vi "newMain.vi"() -> ()   [LabVIEW 2013]
uses:
  <vilib>/NXT/Block Support/NXT_InputPort.ctl
  <vilib>/NXT/Block Support/NXT_OutputPort.ctl
  <vilib>/NXT/Dual Mode Library/Sensors/EV3_Gyro_Reset.vi
  <vilib>/NXT/Dual Mode Library/Sensors/EV3_Ultrasonic_CM.vi
  <vilib>/NXT/NXTIO Xnodes/NXTIONodeSubVIs/NXTStopMotors.vi
  <vilib>/NXT/Subs/LVHSConnector.ctl
  <vilib>/NXT/NXTIO Xnodes/AddressXNode/NXTIOAddress.xnode
  <vilib>/NXT/NXTIO Xnodes/NXTIOXNode/NXTIO.xnode
  <vilib>/NXT/LegoClasses/BrickReference/BrickReference.lvclass
panel:
  out "Numeric 3":dbl
  out "Numeric 2":dbl
  out "Numeric":dbl
  out "isWhite 2":bool
  out "Whiteandblack":bool
  out "blackandwhite":bool
  out "Boolean":bool
  out "to_change":bool
  out "x <= y?":bool
  out "isWhite":bool
  out "isBlack":bool
  out "BlackThenWhite":bool
  out "leftA":dbl
  out "rightB":dbl
  out "identificationWhite":dbl
  out "numOfTargil":dbl
  out "identificationBlack":dbl
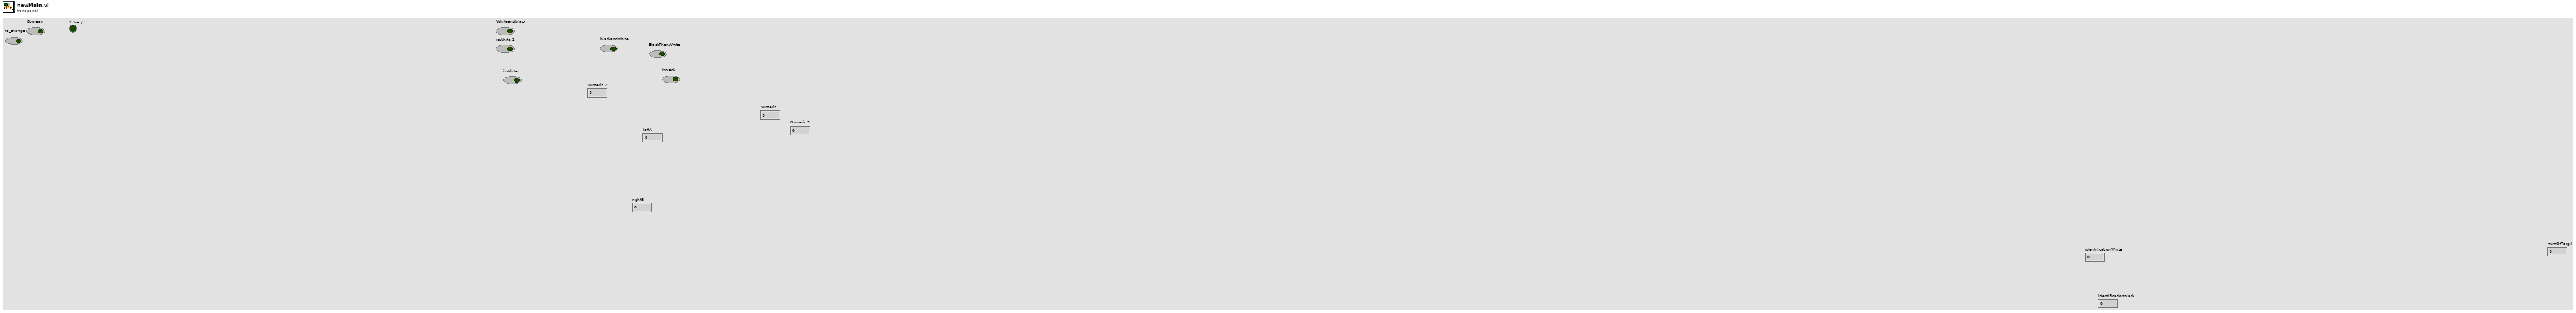
[diagram p1: front panel]
types:
  T1 = typedef "NXT_OutputPort.ctl" = u8
  T2 = typedef "NXT_InputPort.ctl" = u32
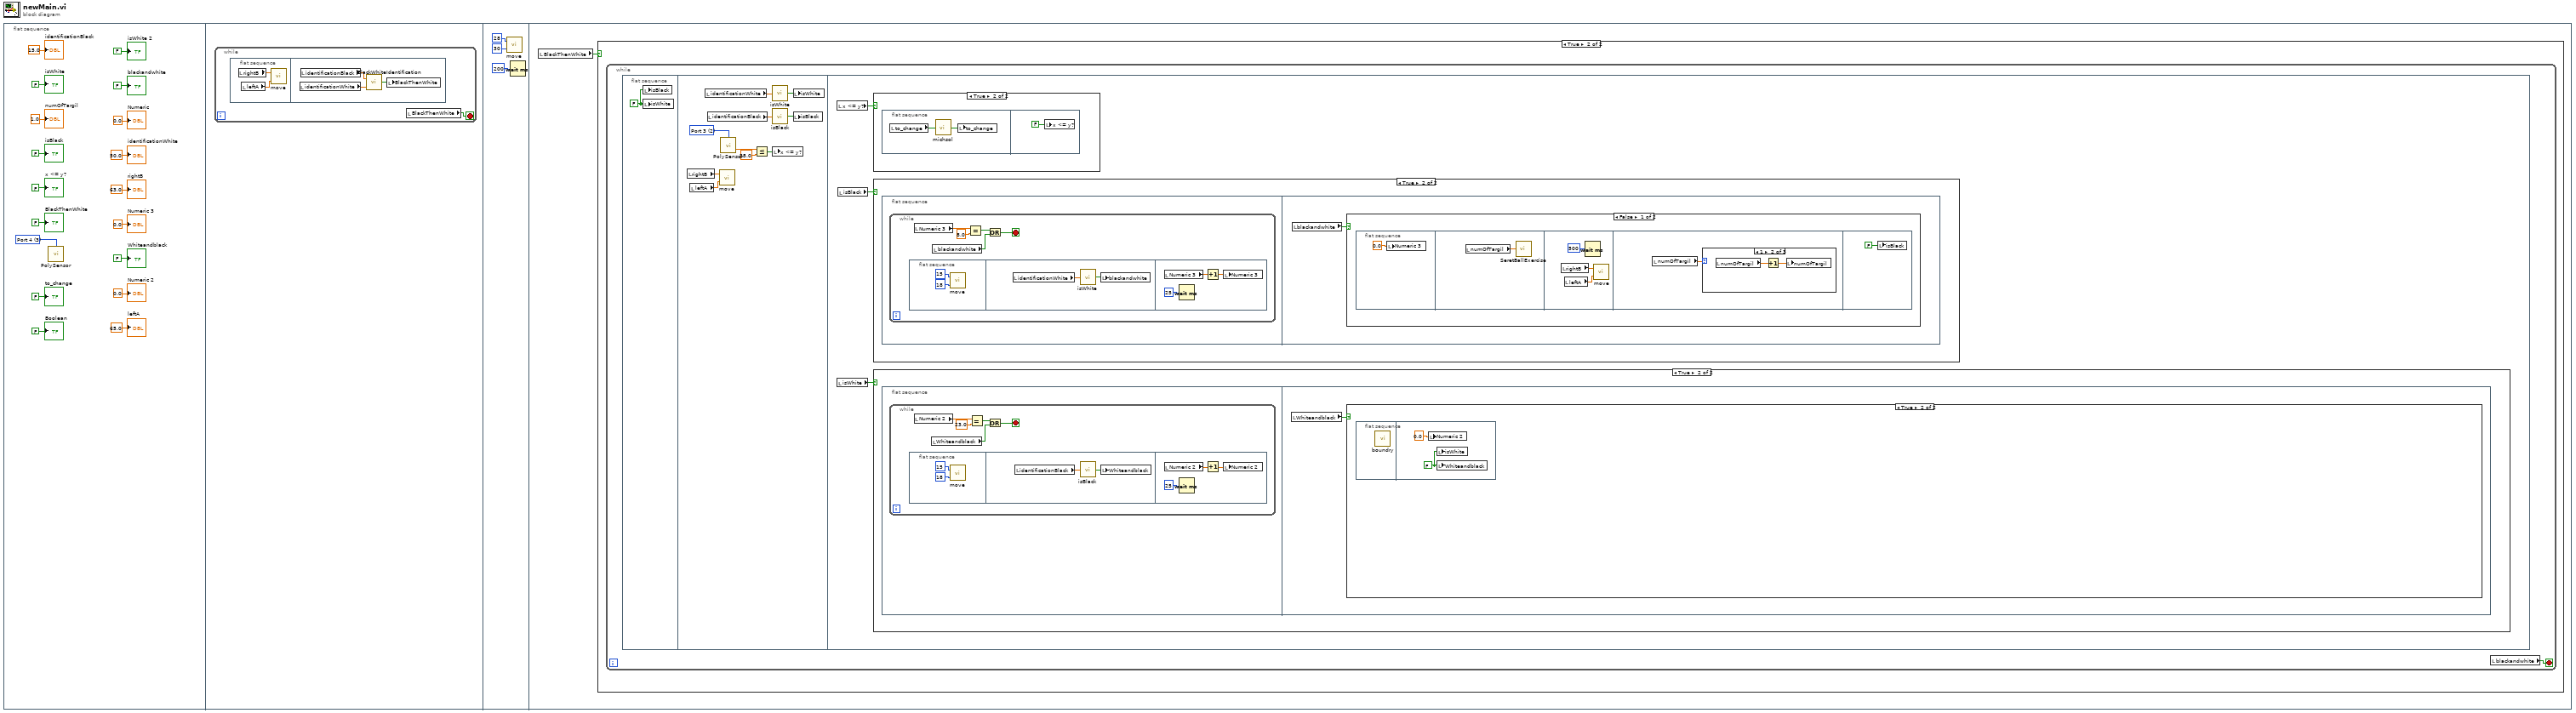
[diagram p0: block diagram]
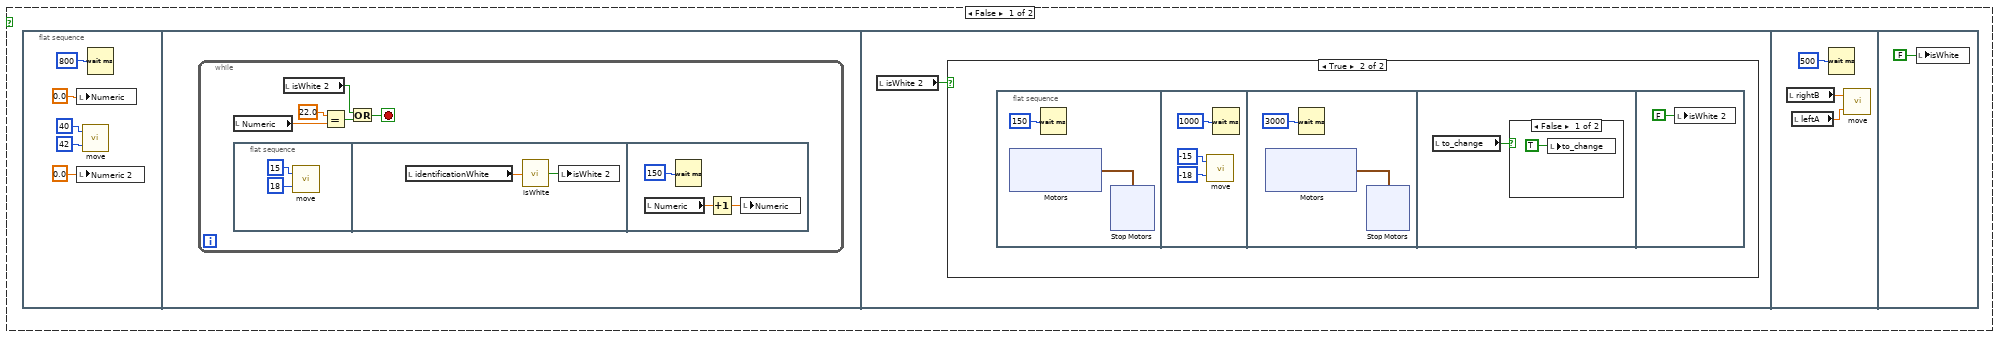
[diagram p4: hidden frame]
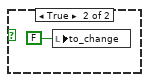
[diagram p6: hidden frame]
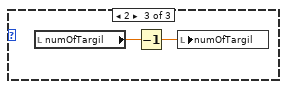
[diagram p9: hidden frame]
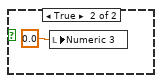
[diagram p10: hidden frame]
diagram:
  n1 = flat-sequence {
    frame #0 {
      w13 = T2 3 items=["Port 1", "Port 2", "Port 3", "Port 4"] ("Port (Port 1)")
      n2 = call-poly <vilib>:"PolySensor.vi"("Port (Port 1)"=w13) -> ()  [unwired: 3 in, 1 out]
      "identificationBlack" <- 15.0 ("identificationBlack")
      "numOfTargil" <- 1.0 ("numOfTargil")
      "identificationWhite" <- 50.0 ("identificationWhite")
      "rightB" <- 63.0 ("Numeric")
      "leftA" <- 65.0 ("leftA")
      "x <= y?" <- FALSE ("x <= y?")
      "isBlack" <- FALSE ("isBlack")
      "isWhite" <- FALSE ("isWhite")
      "to_change" <- FALSE ("Boolean")
      "Boolean" <- FALSE ("Boolean")
      "blackandwhite" <- FALSE ("blackandwhite")
      "Whiteandblack" <- FALSE ("Whiteandblack")
      "BlackThenWhite" <- FALSE ("BlackThenWhite")
      "isWhite 2" <- FALSE ("isWhite 2")
      "Numeric" <- 0.0 ("Numeric")
      "Numeric 2" <- 0.0 ("Numeric 2")
      "Numeric 3" <- 0.0 ("Numeric 3")
    }
    frame #1 {
      n3 = while {
        stop <- w19 stop-if-true
        n4 = flat-sequence {
          frame #0 {
            n5 = local read "rightB"() -> (w20:dbl)
            n6 = local read "leftA"() -> (w21:dbl)
            n7 = call "move.vi"("speedLeft"=w21, "speedRight"=w20) -> ()  [unwired: 1 in]
          }
          frame #1 {
            n8 = local read "identificationWhite"() -> (w23:dbl)
            n9 = local read "identificationBlack"() -> (w24:dbl)
            n10 = call "BlackWhiteIdentification.vi"("whiteBOND"=w23, "BlackBOND"=w24) -> ("BlackThenWhite"=w22:bool)
            n11 = local write "BlackThenWhite"(w22) -> ()
          }
        }
        n12 = local read "BlackThenWhite"() -> (w19:bool)
      }
    }
    frame #2 {
      n13 = call "move.vi"("speedLeft"=i8 30, "speedRight"=i8 28) -> ()  [unwired: 1 in]
      n14 = Wait (ms)(milliseconds to wait=u32 200) -> ()  [unwired: 1 out]
    }
    frame #3 {
      n15 = local read "BlackThenWhite"() -> (w28:bool)
      n16 = case shown="True" w28 {
        frame False {
        }
        frame True {
          n17 = while {
            stop <- w29 stop-if-true
            n18 = flat-sequence {
              frame #0 {
                w30 = FALSE ("isBlack")
                n19 = local write "isBlack"(w30) -> ()
                n20 = local write "isWhite"(w30) -> ()
              }
              frame #1 {
                w39 = T2 2 items=["Port 1", "Port 2", "Port 3", "Port 4"] ("Port (Port 1)")
                n21 = local read "rightB"() -> (w36:dbl)
                n22 = local read "leftA"() -> (w35:dbl)
                n23 = local read "identificationWhite"() -> (w40:dbl)
                n24 = local read "identificationBlack"() -> (w32:dbl)
                n25 = call "move.vi"("speedLeft"=w35, "speedRight"=w36) -> ()  [unwired: 1 in]
                n26 = call-poly <vilib>:"PolySensor.vi"("Port (Port 1)"=w39) -> ("Centimeters"=w38:sgl)  [unwired: 2 in, 1 out]
                n27 = Less Or Equal?(x=w38, y=sgl 35.0) -> (x <= y?=w34:bool)
                n28 = call "isWhite.vi"("whiteBOND"=w40) -> ("isWhite"=w33:bool)
                n29 = call "isBlack.vi"("BlackBOND"=w32) -> ("isBlack"=w31:bool)
                n30 = local write "x <= y?"(w34) -> ()
                n31 = local write "isWhite"(w33) -> ()
                n32 = local write "isBlack"(w31) -> ()
              }
              frame #2 {
                n33 = local read "x <= y?"() -> (w43:bool)
                n34 = local read "isWhite"() -> (w41:bool)
                n35 = local read "isBlack"() -> (w42:bool)
                n36 = case shown="True" w43 {
                  frame False {
                  }
                  frame True {
                    n37 = flat-sequence {
                      frame #0 {
                        n38 = local read "to_change"() -> (w130:bool)
                        n39 = call "michsol.vi"("LEFTOTRETE"=w130) -> ("Boolean"=w129:bool)
                        n40 = local write "to_change"(w129) -> ()
                      }
                      frame #1 {
                        n41 = local write "x <= y?"(FALSE ("x <= y?")) -> ()
                      }
                    }
                  }
                }
                n42 = case shown="True" w42 {
                  frame False {
                  }
                  frame True {
                    n43 = flat-sequence {
                      frame #0 {
                        n44 = while {
                          stop <- w104 stop-if-true
                          n45 = flat-sequence {
                            frame #0 {
                              n46 = call "move.vi"("speedLeft"=i8 18, "speedRight"=i8 15) -> ()  [unwired: 1 in]
                            }
                            frame #1 {
                              n47 = local read "identificationWhite"() -> (w111:dbl)
                              n48 = call "isWhite.vi"("whiteBOND"=w111) -> ("isWhite"=w112:bool)
                              n49 = local write "blackandwhite"(w112) -> ()
                            }
                            frame #2 {
                              n50 = local read "Numeric 3"() -> (w114:dbl)
                              n51 = Wait (ms)(milliseconds to wait=u32 25) -> ()  [unwired: 1 out]
                              n52 = Increment(x=w114) -> (x+1=w115:dbl)
                              n53 = local write "Numeric 3"(w115) -> ()
                            }
                          }
                          n54 = local read "Numeric 3"() -> (w105:dbl)
                          n55 = local read "blackandwhite"() -> (w107:bool)
                          n56 = Equal?(x=w105, y=8.0) -> (x = y?=w106:bool)
                          n57 = Or(x=w106, y=w107) -> (x .or. y?=w104:bool)
                        }
                      }
                      frame #1 {
                        n58 = local read "blackandwhite"() -> (w116:bool)
                        n59 = case shown="False" w116 {
                          frame False {
                            n60 = flat-sequence {
                              frame #0 {
                                n61 = local write "Numeric 3"(0.0 ("Numeric 3")) -> ()
                              }
                              frame #1 {
                                n62 = local read "numOfTargil"() -> (w118:dbl)
                                n63 = call "SeretBallExercise.vi"("ROUND"=w118) -> ()  [unwired: 1 in]
                              }
                              frame #2 {
                                n64 = local read "rightB"() -> (w120:dbl)
                                n65 = local read "leftA"() -> (w119:dbl)
                                n66 = Wait (ms)(milliseconds to wait=u32 500) -> ()  [unwired: 1 out]
                                n67 = call "move.vi"("speedLeft"=w119, "speedRight"=w120) -> ()  [unwired: 1 in]
                              }
                              frame #3 {
                                n68 = local read "numOfTargil"() -> (w122:dbl)
                                n69 = case shown="1" w122 {
                                frame 0, Default {
                                }
                                frame 1 {
                                n70 = local read "numOfTargil"() -> (w124:dbl)
                                n71 = Increment(x=w124) -> (x+1=w123:dbl)
                                n72 = local write "numOfTargil"(w123) -> ()
                                }
                                frame 2 {
                                n73 = local read "numOfTargil"() -> (w126:dbl)
                                n74 = Decrement(x=w126) -> (x-1=w125:dbl)
                                n75 = local write "numOfTargil"(w125) -> ()
                                }
                                }
                              }
                              frame #4 {
                                n76 = local write "isBlack"(FALSE ("isBlack")) -> ()
                              }
                            }
                          }
                          frame True {
                            n77 = local write "Numeric 3"(0.0 ("Numeric 3")) -> ()
                          }
                        }
                      }
                    }
                  }
                }
                n78 = case shown="True" w41 {
                  frame False {
                  }
                  frame True {
                    n79 = flat-sequence {
                      frame #0 {
                        n80 = while {
                          stop <- w45 stop-if-true
                          n81 = flat-sequence {
                            frame #0 {
                              n82 = call "move.vi"("speedLeft"=i8 18, "speedRight"=i8 15) -> ()  [unwired: 1 in]
                            }
                            frame #1 {
                              n83 = local read "identificationBlack"() -> (w52:dbl)
                              n84 = call "isBlack.vi"("BlackBOND"=w52) -> ("isBlack"=w51:bool)
                              n85 = local write "Whiteandblack"(w51) -> ()
                            }
                            frame #2 {
                              n86 = local read "Numeric 2"() -> (w55:dbl)
                              n87 = Wait (ms)(milliseconds to wait=u32 25) -> ()  [unwired: 1 out]
                              n88 = Increment(x=w55) -> (x+1=w54:dbl)
                              n89 = local write "Numeric 2"(w54) -> ()
                            }
                          }
                          n90 = local read "Numeric 2"() -> (w48:dbl)
                          n91 = local read "Whiteandblack"() -> (w46:bool)
                          n92 = Equal?(x=w48, y=23.0) -> (x = y?=w47:bool)
                          n93 = Or(x=w47, y=w46) -> (x .or. y?=w45:bool)
                        }
                      }
                      frame #1 {
                        n94 = local read "Whiteandblack"() -> (w56:bool)
                        n95 = case shown="True" w56 {
                          frame False {
                            n96 = flat-sequence {
                              frame #0 {
                                n97 = local write "Numeric"(0.0 ("Numeric")) -> ()
                                n98 = local write "Numeric 2"(0.0 ("Numeric 2")) -> ()
                                n99 = call "move.vi"("speedLeft"=i8 42, "speedRight"=i8 40) -> ()  [unwired: 1 in]
                                n100 = Wait (ms)(milliseconds to wait=u32 800) -> ()  [unwired: 1 out]
                              }
                              frame #1 {
                                n101 = while {
                                stop <- w65 stop-if-true
                                n102 = local read "Numeric"() -> (w63:dbl)
                                n103 = flat-sequence {
                                frame #0 {
                                n104 = call "move.vi"("speedLeft"=i8 18, "speedRight"=i8 15) -> ()  [unwired: 1 in]
                                }
                                frame #1 {
                                n105 = local read "identificationWhite"() -> (w70:dbl)
                                n106 = call "isWhite.vi"("whiteBOND"=w70) -> ("isWhite"=w69:bool)
                                n107 = local write "isWhite 2"(w69) -> ()
                                }
                                frame #2 {
                                n108 = local read "Numeric"() -> (w73:dbl)
                                n109 = Wait (ms)(milliseconds to wait=u32 150) -> ()  [unwired: 1 out]
                                n110 = Increment(x=w73) -> (x+1=w72:dbl)
                                n111 = local write "Numeric"(w72) -> ()
                                }
                                }
                                n112 = local read "isWhite 2"() -> (w66:bool)
                                n113 = Equal?(x=22.0, y=w63) -> (x = y?=w62:bool)
                                n114 = Or(x=w66, y=w62) -> (x .or. y?=w65:bool)
                                }
                              }
                              frame #2 {
                                n115 = local read "isWhite 2"() -> (w74:bool)
                                n116 = case shown="True" w74 {
                                frame False {
                                }
                                frame True {
                                n117 = flat-sequence {
                                frame #0 {
                                n118 = xnode "Motors"() -> ("Motor"=w76:cluster{"Port":T1, "Port":T1})
                                n119 = Wait (ms)(milliseconds to wait=u32 150) -> ()  [unwired: 1 out]
                                n120 = xnode "Stop Motors"("Motors"=w76) -> ()  [unwired: 1 in, 1 out]
                                }
                                frame #1 {
                                n121 = call "move.vi"("speedLeft"=i8 -18, "speedRight"=i8 -15) -> ()  [unwired: 1 in]
                                n122 = Wait (ms)(milliseconds to wait=u32 1000) -> ()  [unwired: 1 out]
                                }
                                frame #2 {
                                n123 = xnode "Motors"() -> ("Motor"=w87:cluster{"Port":T1, "Port":T1})
                                n124 = Wait (ms)(milliseconds to wait=u32 3000) -> ()  [unwired: 1 out]
                                n125 = xnode "Stop Motors"("Motors"=w87) -> ()  [unwired: 1 in, 1 out]
                                }
                                frame #3 {
                                n126 = local read "to_change"() -> (w94:bool)
                                n127 = case shown="False" w94 {
                                frame False {
                                n128 = local write "to_change"(TRUE ("to_change")) -> ()
                                }
                                frame True {
                                n129 = local write "to_change"(FALSE ("to_change")) -> ()
                                }
                                }
                                }
                                frame #4 {
                                n130 = local write "isWhite 2"(FALSE ("isWhite 2")) -> ()
                                }
                                }
                                }
                                }
                              }
                              frame #3 {
                                n131 = local read "rightB"() -> (w99:dbl)
                                n132 = local read "leftA"() -> (w100:dbl)
                                n133 = Wait (ms)(milliseconds to wait=u32 500) -> ()  [unwired: 1 out]
                                n134 = call "move.vi"("speedLeft"=w100, "speedRight"=w99) -> ()  [unwired: 1 in]
                              }
                              frame #4 {
                                n135 = local write "isWhite"(FALSE ("isWhite")) -> ()
                              }
                            }
                          }
                          frame True {
                            n136 = flat-sequence {
                              frame #0 {
                                n137 = call "boundry.vi"() -> ()  [unwired: 12 in]
                              }
                              frame #1 {
                                w103 = FALSE ("Whiteandblack")
                                n138 = local write "Numeric 2"(0.0 ("Numeric 2")) -> ()
                                n139 = local write "isWhite"(w103) -> ()
                                n140 = local write "Whiteandblack"(w103) -> ()
                              }
                            }
                          }
                        }
                      }
                    }
                  }
                }
              }
            }
            n141 = local read "blackandwhite"() -> (w29:bool)
          }
        }
      }
    }
  }
